vi "GroupSignals.vi"(3 "Signals":T2(array[cluster])) -> (1 "SigGroups":T1(array[cluster]))   [LabVIEW 2024]
panel:
  out "ID Idx Map":map{i32, i32}(c390)
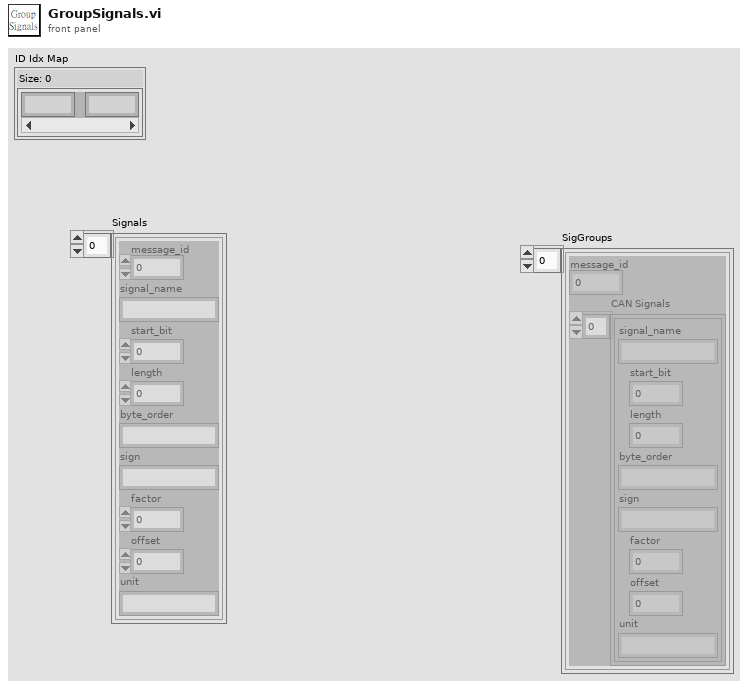
[diagram p1: front panel]
types:
  T1 = cluster{"message_id":i32, "CAN Signals":cluster{"signal_name":string, "start_bit":i32, "length":i32, "byte_order":string, "sign":string, "factor":dbl, "offset":dbl, "unit":string}[]}[]
  T2 = cluster{"message_id":i32, "signal_name":string, "start_bit":i32, "length":i32, "byte_order":string, "sign":string, "factor":dbl, "offset":dbl, "unit":string}[]
  T3 = cluster{"signal_name":string, "start_bit":i32, "length":i32, "byte_order":string, "sign":string, "factor":dbl, "offset":dbl, "unit":string}
  T4 = cluster{"message_id":i32, "CAN Signals":cluster{"signal_name":string, "start_bit":i32, "length":i32, "byte_order":string, "sign":string, "factor":dbl, "offset":dbl, "unit":string}[]}
  T5 = cluster{"signal_name":string, "start_bit":i32, "length":i32, "byte_order":string, "sign":string, "factor":dbl, "offset":dbl, "unit":string}[]
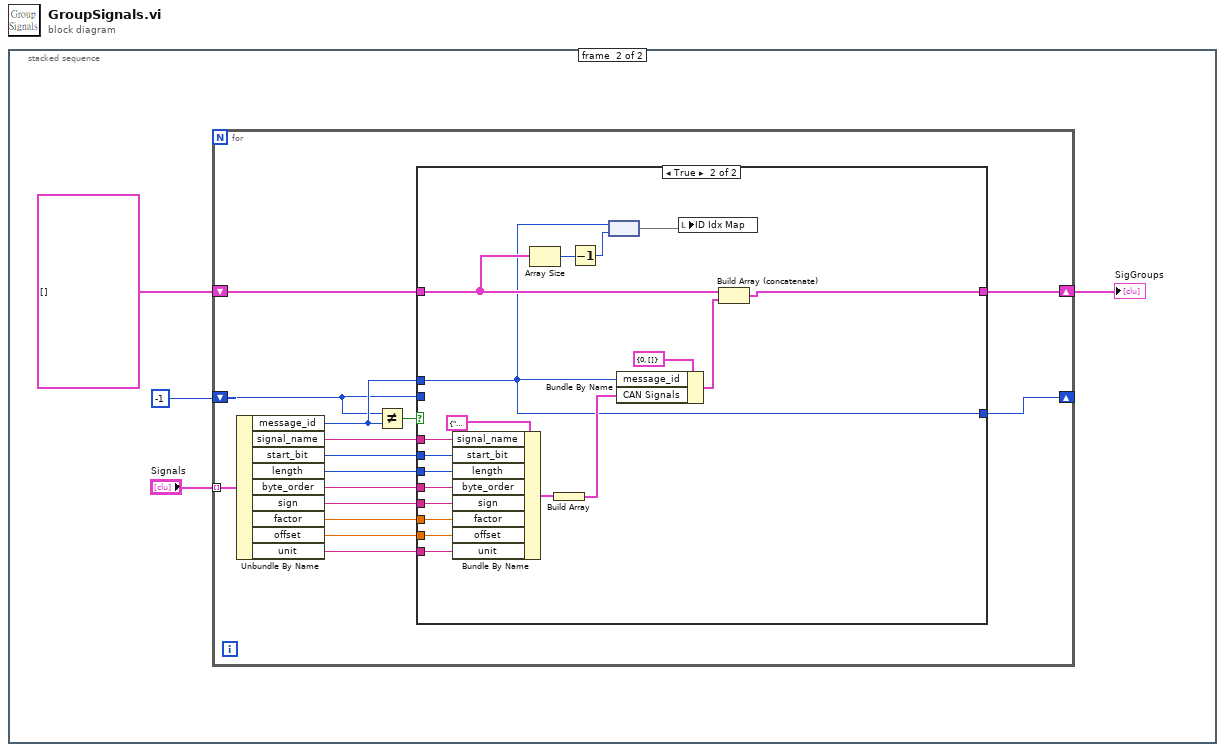
[diagram p0: block diagram]
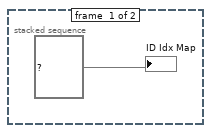
[diagram p2: hidden frame]
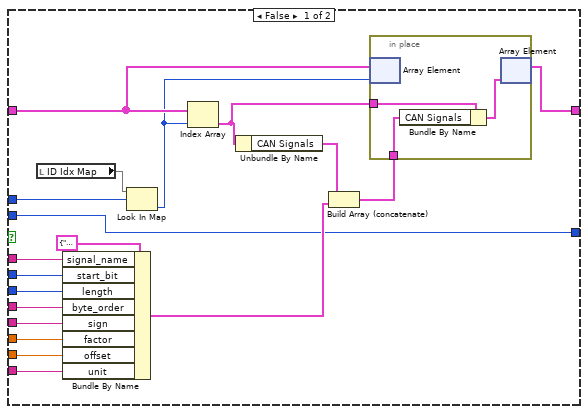
[diagram p3: hidden frame]
diagram:
  n1 = stacked-sequence {
    frame #0 {
      "ID Idx Map" <- map{i32, i32} {} ("ID Idx Map")
    }
    frame #1 {
      n2 = for {
        tunnel: "Signals" -> [w20] mode=indexing
        shift-right: [w7] -> _
        shift-left: -1 -> [w6]
        shift-right: [w8] -> w2
        shift-left: T1 [] ("SigGroups") -> [w9]
        n3 = Unbundle By Name(w20) -> ("message_id"=w10:i32, "signal_name"=w18:string, "start_bit"=w17:i32, "length"=w16:i32, "byte_order"=w15:string, "sign"=w14:string, "factor"=w13:dbl, "offset"=w12:dbl, "unit"=w11:string)
        n4 = Not Equal?(x=w6, y=w10) -> (x != y?=w19:bool)
        n5 = case shown="True" w19 {
          tunnel: w18 -> [w36 w53]
          tunnel: w17 -> [w35 w54]
          tunnel: w16 -> [w34 w55]
          tunnel: w15 -> [w33 w56]
          tunnel: w14 -> [w32 w57]
          tunnel: w13 -> [w31 w58]
          tunnel: w12 -> [w30 w59]
          tunnel: w11 -> [w29 w60]
          tunnel: w10 -> [w38 w43]
          tunnel: w9 -> [w26 w47]
          tunnel: [w22 w48] -> w8
          tunnel: [w21 w43] -> w7
          tunnel: w6 -> [w21 _]
          frame False {
            n6 = local read "ID Idx Map"() -> (w39:map{i32, i32})
            n7 = Bundle By Name(cluster=T3 {"signal_name"="", "start_bit"=0, "length"=0, "byte_order"="", "sign"="", "factor"=0.0, "offset"=0.0, "unit"=""} ("value"), "signal_name"=w36, "start_bit"=w35, "length"=w34, "byte_order"=w33, "sign"=w32, "factor"=w31, "offset"=w30, "unit"=w29) -> (w27:T3)
            n8 = Look In Map(map=w39, key=w38) -> (value=w25:i32)  [unwired: 1 in, 1 out]
            n9 = Index Array(array=w26, index=w25) -> (element=w24:T4)
            n10 = Unbundle By Name(w24) -> ("CAN Signals"=w28:T5)
            n11 = Build Array (concatenate)(w28, w27) -> (w23:T5)
            n12 = in-place {
              in-place-border: w24 -> [w42]
              in-place-border: w23 -> [w41]
              n13 = in-place-array #1(w26, w25) -> ()  [unwired: 1 out]
              n14 = Bundle By Name(cluster=w42, "CAN Signals"=w41) -> (w40:T4)
              n15 = in-place-array #1(w40) -> (w22:T1)  [unwired: 1 out]
            }
          }
          frame True {
            n16 = Bundle By Name(cluster=T3 {"signal_name"="", "start_bit"=0, "length"=0, "byte_order"="", "sign"="", "factor"=0.0, "offset"=0.0, "unit"=""} ("value"), "signal_name"=w53, "start_bit"=w54, "length"=w55, "byte_order"=w56, "sign"=w57, "factor"=w58, "offset"=w59, "unit"=w60) -> (w52:T3)
            n17 = Array Size(array=w47) -> (size(s)=w46:i32)
            n18 = Build Array(w52) -> (w50:T5)
            n19 = Decrement(x=w46) -> (x-1=w45:i32)
            n20 = node(w43, w45) -> (w44:map{i32, i32})
            n21 = Bundle By Name(cluster=T4 {"message_id"=0, "CAN Signals"=[]} ("SignalGroup"), "message_id"=w43, "CAN Signals"=w50) -> (w49:T4)
            n22 = local write "ID Idx Map"(w44) -> ()
            n23 = Build Array (concatenate)(w47, w49) -> (w48:T1)
          }
        }
      }
      "SigGroups" <- w2
    }
  }
